vi "Friendly Name.vi"(8 "error in (no error)":errorcluster, 11 "DeploySerialResource in":refnum<class "SerialResource.lvclass">) -> (0 "error out":errorcluster, 2 "Friendly Name":string, 3 "DeploySerialResource out":refnum<class "SerialResource.lvclass">)   [LabVIEW 2020, in "PicoG-Core.lvlib" / "SerialResource.lvclass"]
uses:
  SerialResource.lvclass
  SerialResource.lvclass/SerialResource.ctl
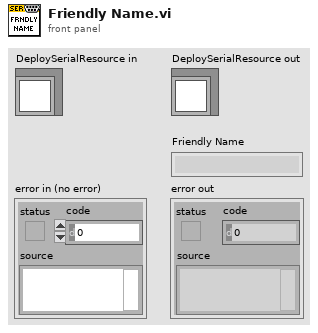
[diagram p1: front panel]
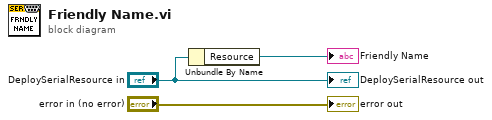
[diagram p0: block diagram]
diagram:
  n1 = Unbundle By Name("DeploySerialResource in") -> ("Resource"=→"Friendly Name":refnum<visa-resource-name>)
  "error out" <- "error in (no error)"
  "DeploySerialResource out" <- "DeploySerialResource in"
